vi "Get Command Infos.vi"(8 "error in (no error)":errorcluster, 11 "Mouse in":refnum<class "Mouse.lvclass">) -> (0 "error out":errorcluster, 3 "Mouse out":refnum<class "Mouse.lvclass">, 4 "Direction info out":string, 6 "Boost info out":string)   [LabVIEW 2021, in "Mouse.lvclass"]
doc: "MIT Licence\nCopyright (c) 2024 David Grollier"
uses:
  Mouse.lvclass
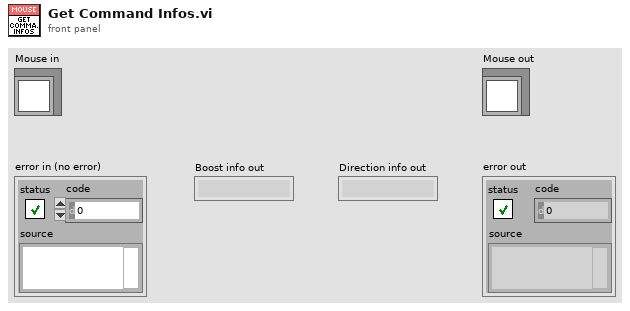
[diagram p1: front panel]
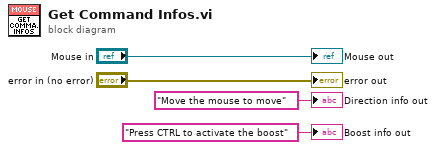
[diagram p0: block diagram]
diagram:
  "error out" <- "error in (no error)"
  "Mouse out" <- "Mouse in"
  "Direction info out" <- "Move the mouse to move" ("Direction info out")
  "Boost info out" <- "Press CTRL to activate the boost" ("Boost info out")
